vi "Enqueue Message.vi"(6 "Priority?":bool, 7 "Flush?":bool, 8 "error in (no error)":errorcluster, 9 "Data":variant, 10 "State":T1, 11 "queue in":refnum<queue>) -> (0 "error out":errorcluster, 3 "queue out":refnum<queue>)   [LabVIEW 2021, in "Queue Library.lvlib"]
uses:
  Queue Library.lvlib
  Controls/Message.ctl
  Controls/State.ctl
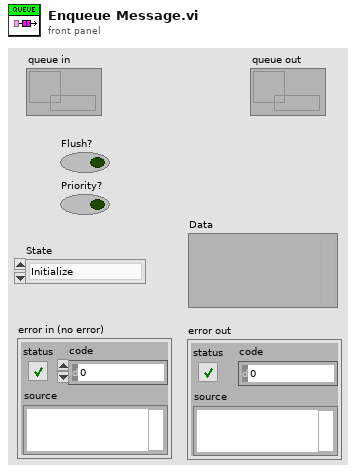
[diagram p1: front panel]
types:
  T1 = typedef "State.ctl" = enum16{"Initialize", "Idle", "Start Scope", "Acquire", "Stop Scope", "Config FGen", "Start FGen", "Sweep FGen", "Stop FGen", "Plot", "Option Selection", "Channel 0 Selection", "Channel 1 Selection", "Update Cursors", "Update Measurements", "Time/Div", "Autoscale", "Stop", "Error"}
  T2 = typedef "Message.ctl" = cluster{"State":T1, "Data":variant}
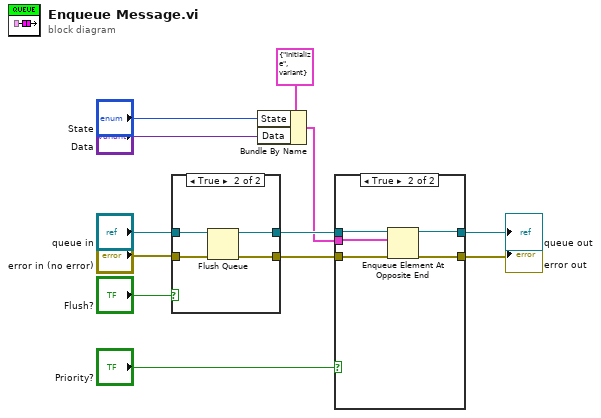
[diagram p0: block diagram]
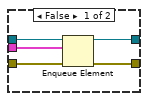
[diagram p2: hidden frame]
diagram:
  n1 = case shown="True" "Flush?" {
    tunnel: "queue in" -> [w14 w18]
    tunnel: "error in (no error)" -> [w13 w17]
    tunnel: [w14 w16] -> w8
    tunnel: [w13 w15] -> w7
    frame False {
    }
    frame True {
      n2 = Flush Queue(queue=w18, error in (no error)=w17) -> (queue out=w16:refnum<queue>, error out=w15:errorcluster)  [unwired: 1 out]
    }
  }
  n3 = Bundle By Name(cluster=T2 {"State"=enum."Initialize", "Data"=variant} ("element"), "State"="State", "Data"="Data") -> (w3:T2)
  n4 = case shown="True" "Priority?" {
    tunnel: w8 -> [w23 w28]
    tunnel: w7 -> [w22 w27]
    tunnel: [w21 w26] -> w6
    tunnel: [w20 w25] -> w5
    tunnel: w3 -> [w19 w24]
    frame False {
      n5 = Enqueue Element(queue=w23, element=w19, error in (no error)=w22) -> (queue out=w21:refnum<queue>, error out=w20:errorcluster)  [unwired: 1 in, 1 out]
    }
    frame True {
      n6 = Enqueue Element At Opposite End(queue=w28, element=w24, error in (no error)=w27) -> (queue out=w26:refnum<queue>, error out=w25:errorcluster)  [unwired: 1 in, 1 out]
    }
  }
  "queue out" <- w6
  "error out" <- w5
